vi "Read Process SV.vi"(8 "error in (no error)":errorcluster, 11 "EMKO in":refnum<class "ESM-xx50.lvclass">) -> (0 "error out":errorcluster, 2 "Process SV":u16, 3 "EMKO out":refnum<class "ESM-xx50.lvclass">)   [LabVIEW 2022 SP3, in "EMKO.lvlib" / "ESM-xx50.lvclass"]
uses:
  ESM-xx50.lvclass
  ESM-xx50.lvclass/ESM-xx50.ctl
  <vilib>/Modbus/master/Modbus Master.lvclass
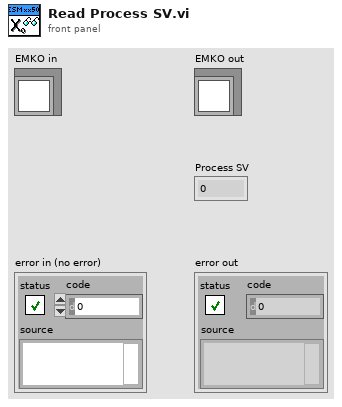
[diagram p1: front panel]
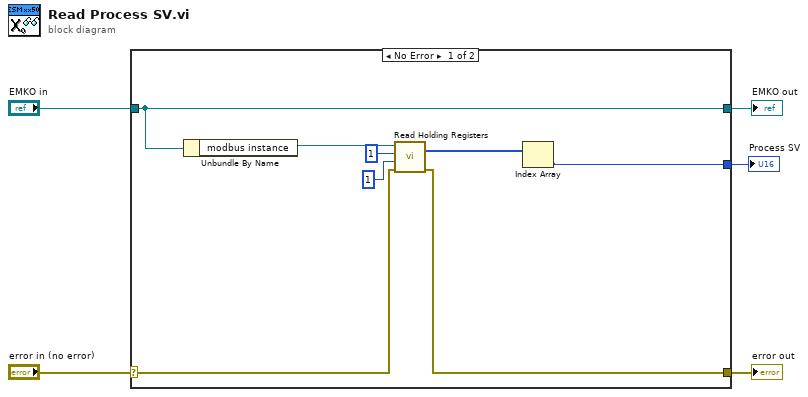
[diagram p0: block diagram]
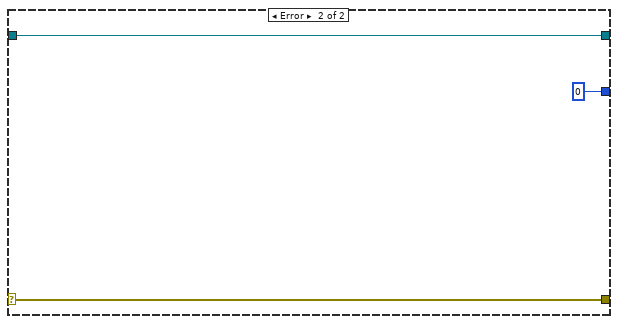
[diagram p2: hidden frame]
diagram:
  n1 = case shown="No Error" "error in (no error)" {
    selector: "error in (no error)" -> [w9 w16]
    tunnel: [w8 w16] -> w4
    tunnel: [w13 w15] -> w2
    tunnel: "EMKO in" -> [w13 w15]
    tunnel: [w6 u16 0 ("register")] -> w1
    frame No Error {
      n2 = Unbundle By Name(w13) -> ("modbus instance"=w12:refnum<class "Modbus Master.lvclass">)
      n3 = call-dynamic "Read Holding Registers.vi"("error in (no error)"=w9, "number of holding registers"=u16 1, "starting address"=u16 1, "Modbus master in"=w12) -> ("error out"=w8:errorcluster, "register values"=w7:u16[])  [unwired: 5 in, 1 out]
      n4 = Index Array(array=w7) -> (element=w6:u16)  [unwired: 1 in]
    }
    frame Error {
    }
  }
  "error out" <- w4
  "EMKO out" <- w2
  "Process SV" <- w1
